vi "Set Packet Message Reference.vi"(10 "Packet Msg":refnum<class "Packet Msg.lvclass">, 11 "TCPIP Communications in":refnum<class "TCPIP Communications.lvclass">) -> (3 "TCPIP Communications out":refnum<class "TCPIP Communications.lvclass">)   [LabVIEW 2015, in "TCPIP Communications Framework.lvlib" / "TCPIP Communications.lvclass"]
uses:
  TCPIP Communications.lvclass
  TCPIP Communications Messages/Packet Msg/Packet Msg.lvclass
  TCPIP Communications.lvclass/TCPIP Communications.ctl
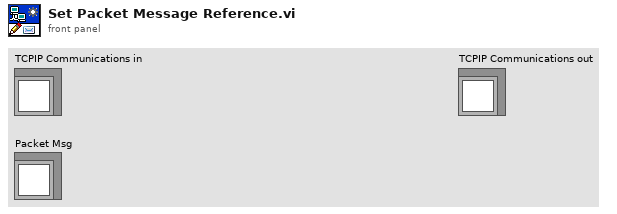
[diagram p1: front panel]
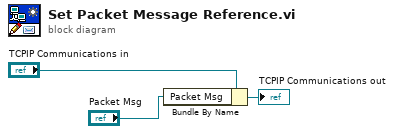
[diagram p0: block diagram]
diagram:
  n1 = Bundle By Name(cluster="TCPIP Communications in", "Packet Msg"="Packet Msg") -> (→"TCPIP Communications out":refnum<class "TCPIP Communications.lvclass">)
